vi "calculate_abs.vi"(10 "RMS":dbl[](array[numeric]), 11 "measured_value":dbl[](array[numeric])) -> (3 "Array":dbl[](array[numeric]))   [LabVIEW 2017]
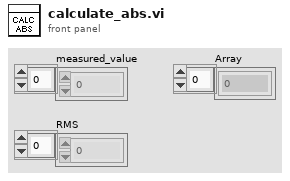
[diagram p1: front panel]
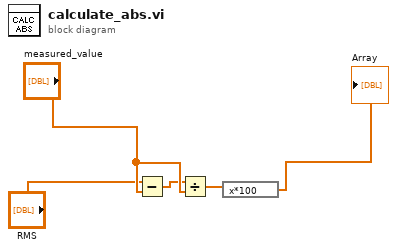
[diagram p0: block diagram]
diagram:
  n1 = Subtract(x="RMS", y="measured_value") -> (x-y=w2:dbl[])
  n2 = Divide(x=w2, y="measured_value") -> (x/y=w4:dbl[])
  n3 = expression code="x*100"(w4) -> (→"Array":dbl[])
